vi "Analog Channel Select v2.0 (SubVI).vi"() -> (0 "error out":errorcluster, 1 "task out":refnum<k21>, 2 "samples per channel":i32=1)   [LabVIEW 2020]
uses:
  <vilib>/DAQmx/create/channels.llb/DAQmx Create Channel (AI-Voltage-Basic).vi
  <vilib>/DAQmx/create/channels.llb/DAQmx Create Channel (TEDS-AI-Voltage-Basic).vi
  <vilib>/DAQmx/create/channels.llb/DAQmx Create Channel (AI-Temperature-Thermocouple).vi
  <vilib>/DAQmx/configure/timing.llb/DAQmx Timing (Sample Clock).vi
  <resource>/objmgr/daqmx.rc
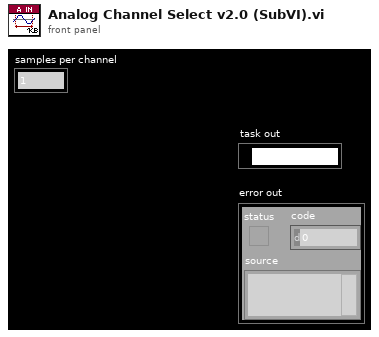
[diagram p1: front panel]
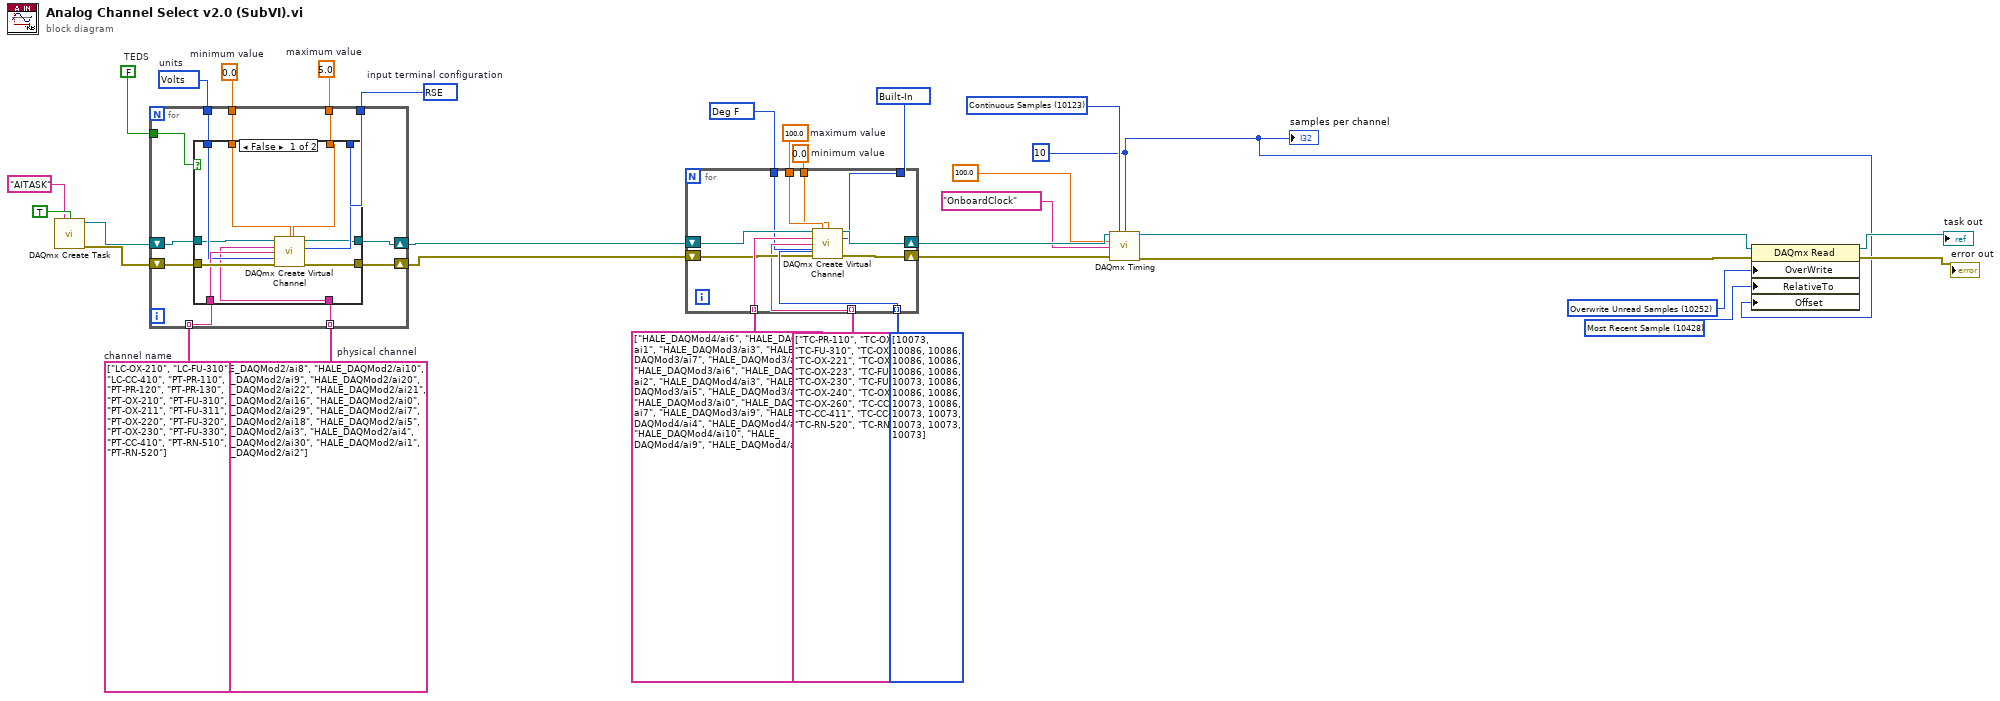
[diagram p0: block diagram]
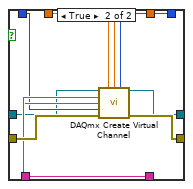
[diagram p2: hidden frame]
diagram:
  w3 = 10 ("samples per channel 2")
  w6 = 10428 items=["First Sample"=10424, "Current Read Position"=10425, "Reference Trigger"=10426, "First Pretrigger Sample"=10427, "Most Recent Sample"=10428] ("RelativeTo")
  w7 = 10252 items=["Overwrite Unread Samples"=10252, "Do Not Overwrite Unread Samples"=10159] ("OverWrite")
  w9 = 10123 items=["Finite Samples"=10178, "Continuous Samples"=10123, "Hardware Timed Single Point"=12522] ("sample mode")
  w30 = 10200 items=["Built-In"=10200, "Constant Value"=10116, "Channel"=10113] ("cjc source")
  w31 = 0.0  # minimum value
  w32 = 100.0  # maximum value
  w28 = 10144 items=["Deg C"=10143, "Deg F"=10144, "Kelvins"=10325, "Deg R"=10145, "From Custom Scale"=10065] ("units")
  w26 = i32[] [10073, 10086, 10086, 10086, 10086, 10086, 10086, 10073, 10086, 10086, 10086, 10073, 10086, 10073, 10073, 10073, 10073, 10073] items=["J"=10072, "K"=10073, "N"=10077, "R"=10082, "S"=10085, "T"=10086, "B"=10047, "E"=10055] ("thermocouple type")
  w20 = 5.0  # maximum value
  w21 = 0.0  # minimum value
  w18 = FALSE  # TEDS
  w17 = 10348 items=["Volts"=10348, "From TEDS"=12516, "From Custom Scale"=10065]  # units
  w19 = string[] ["LC-OX-210", "LC-FU-310", "LC-CC-410", "PT-PR-110", "PT-PR-120", "PT-PR-130", "PT-OX-210", "PT-FU-310", "PT-OX-211", "PT-FU-311", "PT-OX-220", "PT-FU-320", "PT-OX-230", "PT-FU-330", "PT-CC-410", "PT-RN-510", "PT-RN-520"]  # channel name
  w16 = 10083 items=["default"=-1, "RSE"=10083, "NRSE"=10078, "Differential"=10106, "Pseudodifferential"=12529]  # input terminal configuration
  w15 = tag[] ["HALE_DAQMod2/ai8", "HALE_DAQMod2/ai10", "HALE_DAQMod2/ai9", "HALE_DAQMod2/ai20", "HALE_DAQMod2/ai22", "HALE_DAQMod2/ai21", "HALE_DAQMod2/ai16", "HALE_DAQMod2/ai0", "HALE_DAQMod2/ai29", "HALE_DAQMod2/ai7", "HALE_DAQMod2/ai18", "HALE_DAQMod2/ai5", "HALE_DAQMod2/ai3", "HALE_DAQMod2/ai4", "HALE_DAQMod2/ai30", "HALE_DAQMod2/ai1", "HALE_DAQMod2/ai2"]  # physical channel
  n1 = call <vilib>:"DAQmx Create Task.vi"("new task name"="AITASK", "auto cleanup"=TRUE) -> ("task out"=w23:refnum<k21>, "error out"=w25:errorcluster)  [unwired: 12 in]
  n2 = for {
    tunnel: w16 -> [w33]
    tunnel: w21 -> [w42]
    tunnel: w20 -> [w43]
    tunnel: w17 -> [w37]
    tunnel: w19 -> [w39] mode=indexing
    tunnel: w15 -> [w38] mode=indexing
    shift-right: [w40] -> w14
    shift-left: w25 -> [w41]
    tunnel: w18 -> [w36]
    shift-right: [w34] -> w8
    shift-left: w23 -> [w35]
    n3 = case shown="False" w36 {
      tunnel: w43 -> [w53 w59]
      tunnel: w42 -> [w44 w60]
      tunnel: w33 -> [w52 w61]
      tunnel: w41 -> [w51 w63]
      tunnel: [w50 w62] -> w40
      tunnel: w39 -> [w49 w57]
      tunnel: w38 -> [w47 w58]
      tunnel: w37 -> [w48 w56]
      tunnel: w35 -> [w45 w54]
      tunnel: [w46 w55] -> w34
      frame False {
        n4 = call-poly <vilib>:"DAQmx Create Virtual Channel.vi"("task in"=w45, "maximum value"=w53, "minimum value"=w44, "input terminal configuration"=w52, "physical channels"=w47, "name to assign"=w49, "units"=w48, "error in"=w51) -> ("task out"=w46:refnum<k21>, "error out"=w50:errorcluster)  [unwired: 6 in]
      }
      frame True {
        n5 = call-poly <vilib>:"DAQmx Create Virtual Channel.vi"("task in"=w54, "maximum value"=w59, "minimum value"=w60, "input terminal configuration"=w61, "physical channels"=w58, "name to assign"=w57, "units"=w56, "error in"=w63) -> ("task out"=w55:refnum<k21>, "error out"=w62:errorcluster)  [unwired: 6 in]
      }
    }
  }
  n6 = for {
    tunnel: tag[] ["HALE_DAQMod4/ai6", "HALE_DAQMod3/ai1", "HALE_DAQMod3/ai3", "HALE_DAQMod3/ai7", "HALE_DAQMod3/ai4", "HALE_DAQMod3/ai6", "HALE_DAQMod3/ai2", "HALE_DAQMod4/ai3", "HALE_DAQMod3/ai5", "HALE_DAQMod3/ai8", "HALE_DAQMod3/ai0", "HALE_DAQMod4/ai7", "HALE_DAQMod3/ai9", "HALE_DAQMod4/ai4", "HALE_DAQMod4/ai5", "HALE_DAQMod4/ai10", "HALE_DAQMod4/ai9", "HALE_DAQMod4/ai8"] ("physical channels") -> [w74] mode=indexing
    tunnel: w26 -> [w73] mode=indexing
    shift-right: [w72] -> w13
    shift-left: w8 -> [w70]
    shift-right: [w71] -> w12
    shift-left: w14 -> [w69]
    tunnel: string[] ["TC-PR-110", "TC-OX-210", "TC-FU-310", "TC-OX-220", "TC-OX-221", "TC-OX-222", "TC-OX-223", "TC-FU-320", "TC-OX-230", "TC-FU-330", "TC-OX-240", "TC-OX-250", "TC-OX-260", "TC-CC-410", "TC-CC-411", "TC-CC-412", "TC-RN-520", "TC-RN-530"] ("name to assign") -> [w68] mode=indexing
    tunnel: w32 -> [w67]
    tunnel: w31 -> [w66]
    tunnel: w30 -> [w65]
    tunnel: w28 -> [w64]
    n7 = call-poly <vilib>:"DAQmx Create Virtual Channel.vi"("task in"=w70, "maximum value"=w67, "minimum value"=w66, "physical channels"=w74, "cjc source"=w65, "name to assign"=w68, "units"=w64, "error in"=w69, "thermocouple type"=w73) -> ("task out"=w72:refnum<k21>, "error out"=w71:errorcluster)  [unwired: 5 in]
  }
  n8 = call-poly <vilib>:"DAQmx Timing.vi"("task/channels in"=w13, "sample mode"=w9, "samples per channel"=w3, "rate"=100.0, "source"=tag "OnboardClock", "error in"=w12) -> ("task out"=w2:refnum<k21>, "error out"=w1:errorcluster)  [unwired: 8 in]
  n9 = property class="DAQmx Read"(reference=w2, error in=w1, "OverWrite"=w7, "RelativeTo"=w6, "Offset"=w3) -> (reference out=→"task out":refnum<k21>, error out=→"error out":errorcluster)
  "samples per channel" <- w3
